vi "Experiment header-update fgv internal params.vi"(8 "error in (no error)":errorcluster, 10 "All header parameters in":T1={"LOGIN"={"User"="Olympus  20X", "Profile"="", "Software Version"="", "Experiment Date Time"=timestamp(0 s since 1904-01-01)}, "GLOBAL PARAMETERS"={"MicroscopeID"="", "Microscope Type"="", "Objective"="", "Field of View (um)"=0.0, "Fill time (us)"=0.0, "Experiment Type"=enum."In vivo", "Stimuli Trigger"=FALSE, "Speed Logging"=FALSE}, "IMAGING MODES"={"Time Series"=FALSE, "Motor Zstack"=FALSE, "AOL Zstack"=FALSE, "Functional Imaging"=FALSE, "Volume Imaging"=FALSE}, "TIME SERIES"={"Basic Image meta data"={"Wavelength (nm)"=0.0, "# averaged frames"=0.0, "laser power (%)"=0.0, "Pockels"=0.0, "pixel dwell time (us)"=0.0, "pmt 1"=0.0, "pmt 2"=0.0, "back apperture"=0.0, "zoom"=0.0, "field of view"=0.0, "Frame Size"=0, "AOL x centre"=0.0, "AOL y centre"=0.0, "Stage x position"=0.0, "Stage y position"=0.0, "Stage z position"=0.0}, "AOL z"=0.0}, "MOTOR Z-STACK "={"Hdr Basic Image meta data"={"Wavelength (nm)"=0.0, "# averaged frames"=0.0, "laser power (%)"=0.0, "Pockels"=0.0, "pixel dwell time (us)"=0.0, "pmt 1"=0.0, "pmt 2"=0.0, "back apperture"=0.0, "zoom"=0.0, "field of view"=0.0, "Frame Size"=0, "AOL x centre"=0.0, "AOL y centre"=0.0, "Stage x position"=0.0, "Stage y position"=0.0, "Stage z position"=0.0}, "Z Start"=0.0, "Z Stop"=0.0, "No of Planes"=0}, "AOL Z-STACK"={"Hdr Basic Image meta data"={"Wavelength (nm)"=0.0, "# averaged frames"=0.0, "laser power (%)"=0.0, "Pockels"=0.0, "pixel dwell time (us)"=0.0, "pmt 1"=0.0, "pmt 2"=0.0, "back apperture"=0.0, "zoom"=0.0, "field of view"=0.0, "Frame Size"=0, "AOL x centre"=0.0, "AOL y centre"=0.0, "Stage x position"=0.0, "Stage y position"=0.0, "Stage z position"=0.0}, "Z Start"=0.0, "Z Stop"=0.0, "No of Planes"=0}, "FUNCTIONAL IMAGING"={"Functional Mode"=enum."Point", "Pockels Modulation"=FALSE, "Number of pois"=0.0, "Number of miniscans"=0.0, "Number of cycles"=0.0, "Number of trials"=0.0, "Miniscan dwell time per pixel (us)"=0.0, "Number of pixels in miniscan"=0.0, "poi dwell time"=0.0, "Rectangle ROI length"=0.0, "Rectangle ROI height"=0.0, "AOL Mode"=enum."Raster", "Plane Mode"=0, "video length (sec)"=0.0, "Frame rate (fps)"=0.0, "Stimuli Timing (usec)"=0.0, "Acquisition Length"=0.0, "Basic Image meta data"={"Wavelength (nm)"=0.0, "# averaged frames"=0.0, "laser power (%)"=0.0, "Pockels"=0.0, "pixel dwell time (us)"=0.0, "pmt 1"=0.0, "pmt 2"=0.0, "back apperture"=0.0, "zoom"=0.0, "field of view"=0.0, "Frame Size"=0, "AOL x centre"=0.0, "AOL y centre"=0.0, "Stage x position"=0.0, "Stage y position"=0.0, "Stage z position"=0.0}, "Z Start (um)"=0.0, "Z Stop (um)"=0.0}, "VOLUME IMAGING"={"Functional Mode"=enum."Point", "Pockels Modulation"=FALSE, "Number of pois"=0.0, "Number of miniscans"=0.0, "Number of cycles"=0.0, "Number of trials"=0.0, "Miniscan dwell time per pixel (us)"=0.0, "Number of pixels in miniscan"=0.0, "poi dwell time"=0.0, "Rectangle ROI length"=0.0, "Rectangle ROI height"=0.0, "AOL Mode"=enum."Raster", "Plane Mode"=0, "video length (sec)"=0.0, "Frame rate (fps)"=0.0, "Stimuli Timing (usec)"=0.0, "Acquisition Length"=0.0, "Basic Image meta data"={"Wavelength (nm)"=0.0, "# averaged frames"=0.0, "laser power (%)"=0.0, "Pockels"=0.0, "pixel dwell time (us)"=0.0, "pmt 1"=0.0, "pmt 2"=0.0, "back apperture"=0.0, "zoom"=0.0, "field of view"=0.0, "Frame Size"=0, "AOL x centre"=0.0, "AOL y centre"=0.0, "Stage x position"=0.0, "Stage y position"=0.0, "Stage z position"=0.0}, "Z Start (um)"=0.0, "Z Stop (um)"=0.0}, "MOVEMENT CORRECTION"={"Movement Correction"=FALSE, "Axial Reference"=FALSE, "Reference X Pixels"=0.0, "Reference Y Pixels"=0.0, "Reference Source"=enum."Green channel", "Reference dwell time (us)"=0.0, "Number of Z lines"=0.0, "Size of Z pixels"=0.0, "Axial Pixels"=0.0, "Reference Zoom"=0.0, "Reference Average"=0.0, "Proportional Scale"=0.0, "Integral Scale"=0.0, "Proportional Scale Z"=0.0, "Integral Scale Z"=0.0, "Scan Interval"=0.0, "Ref Plot Refresh Rate"=0.0}, "CALIBRATION"={"Pockels Calibration File"=path "", "Calibration_ini file"=path "", "Setup_ini file"=path ""}, "STATISTICS"={"Z-stack duration (sec)"=0.0, "Number of acquired data-points"=0.0, "Acquisition time (ms)"=0.0, "Number of acquired frames"=0.0}, "BIOLOGY INFORMATION"={"Animal Code or Name"="", "Animal DoB"="", "Animal Age"="", "Animal Sex"="", "Animal Weight"="", "Date of Injection"="", "Date of Implant"="", "Site of Injection"="", "Animal Ear Notch"="", "AAV constructs"="", "Genetic background"="", "Optical reporter"="", "Region of brain imaged"="", "Other \ncomments"=""}} {"VOLUME IMAGING"."Plane Mode" items=["XY Plane", "XZ Plane", "YZ Plane", "arbitraryplane"]; "VOLUME IMAGING"."Basic Image meta data"."Frame Size" items=["100X100"=100, "128X128"=128, "200X200"=200, "256X256"=256, "512X512"=512, "1024x1024"=1024, "2048x2048"=2048]; "AOL Z-STACK"."Hdr Basic Image meta data"."Frame Size" items=["100X100"=100, "128X128"=128, "200X200"=200, "256X256"=256, "512X512"=512, "1024x1024"=1024, "2048x2048"=2048]; "MOTOR Z-STACK"."Hdr Basic Image meta data"."Frame Size" items=["100X100"=100, "128X128"=128, "200X200"=200, "256X256"=256, "512X512"=512, "1024x1024"=1024, "2048x2048"=2048]; "FUNCTIONAL IMAGING"."Plane Mode" items=["XY Plane", "XZ Plane", "YZ Plane", "arbitraryplane"]; "FUNCTIONAL IMAGING"."Basic Image meta data"."Frame Size" items=["100X100"=100, "128X128"=128, "200X200"=200, "256X256"=256, "512X512"=512, "1024x1024"=1024, "2048x2048"=2048]; "TIME SERIES"."Basic Image meta data"."Frame Size" items=["100X100"=100, "128X128"=128, "200X200"=200, "256X256"=256, "512X512"=512, "1024x1024"=1024, "2048x2048"=2048]}, 11 "All header parameters / Header module interface cluster":refnum<vi>) -> (0 "error out":errorcluster, 3 "All header parameters OUT":refnum<vi>)   [LabVIEW 2017]
uses:
  Typedefs/Header parameters cluster-ALL.ctl
  Typedefs/Header subclusters/Header params -Login.ctl
  Typedefs/Header subclusters/Header params-Global Parameters.ctl
  Misc/Experiment Type.ctl
  Typedefs/Header subclusters/Header params-Imaging Modes.ctl
  Typedefs/Header subclusters/Header params-Time Series.ctl
  Typedefs/Header subclusters/Header params-Basic image meta data.ctl
  Typedefs/Frame Size.ctl
  Typedefs/Header subclusters/Header params-Motor Z-stack.ctl
  Typedefs/Header subclusters/Header params-AOL Z-stack.ctl
  Typedefs/Header subclusters/Header params-Functional Imaging.ctl
  Typedefs/Functional Mode.ctl
  Typedefs/AOL modes.ctl
  Typedefs/Plane Mode.ctl
  Typedefs/Header subclusters/Header params-Movement correction.ctl
  Typedefs/Reference source.ctl
  Typedefs/Header subclusters/Header params-Calibration Setup.ctl
  Typedefs/Header subclusters/Header params-statistics.ctl
  Misc/Biology Information.ctl
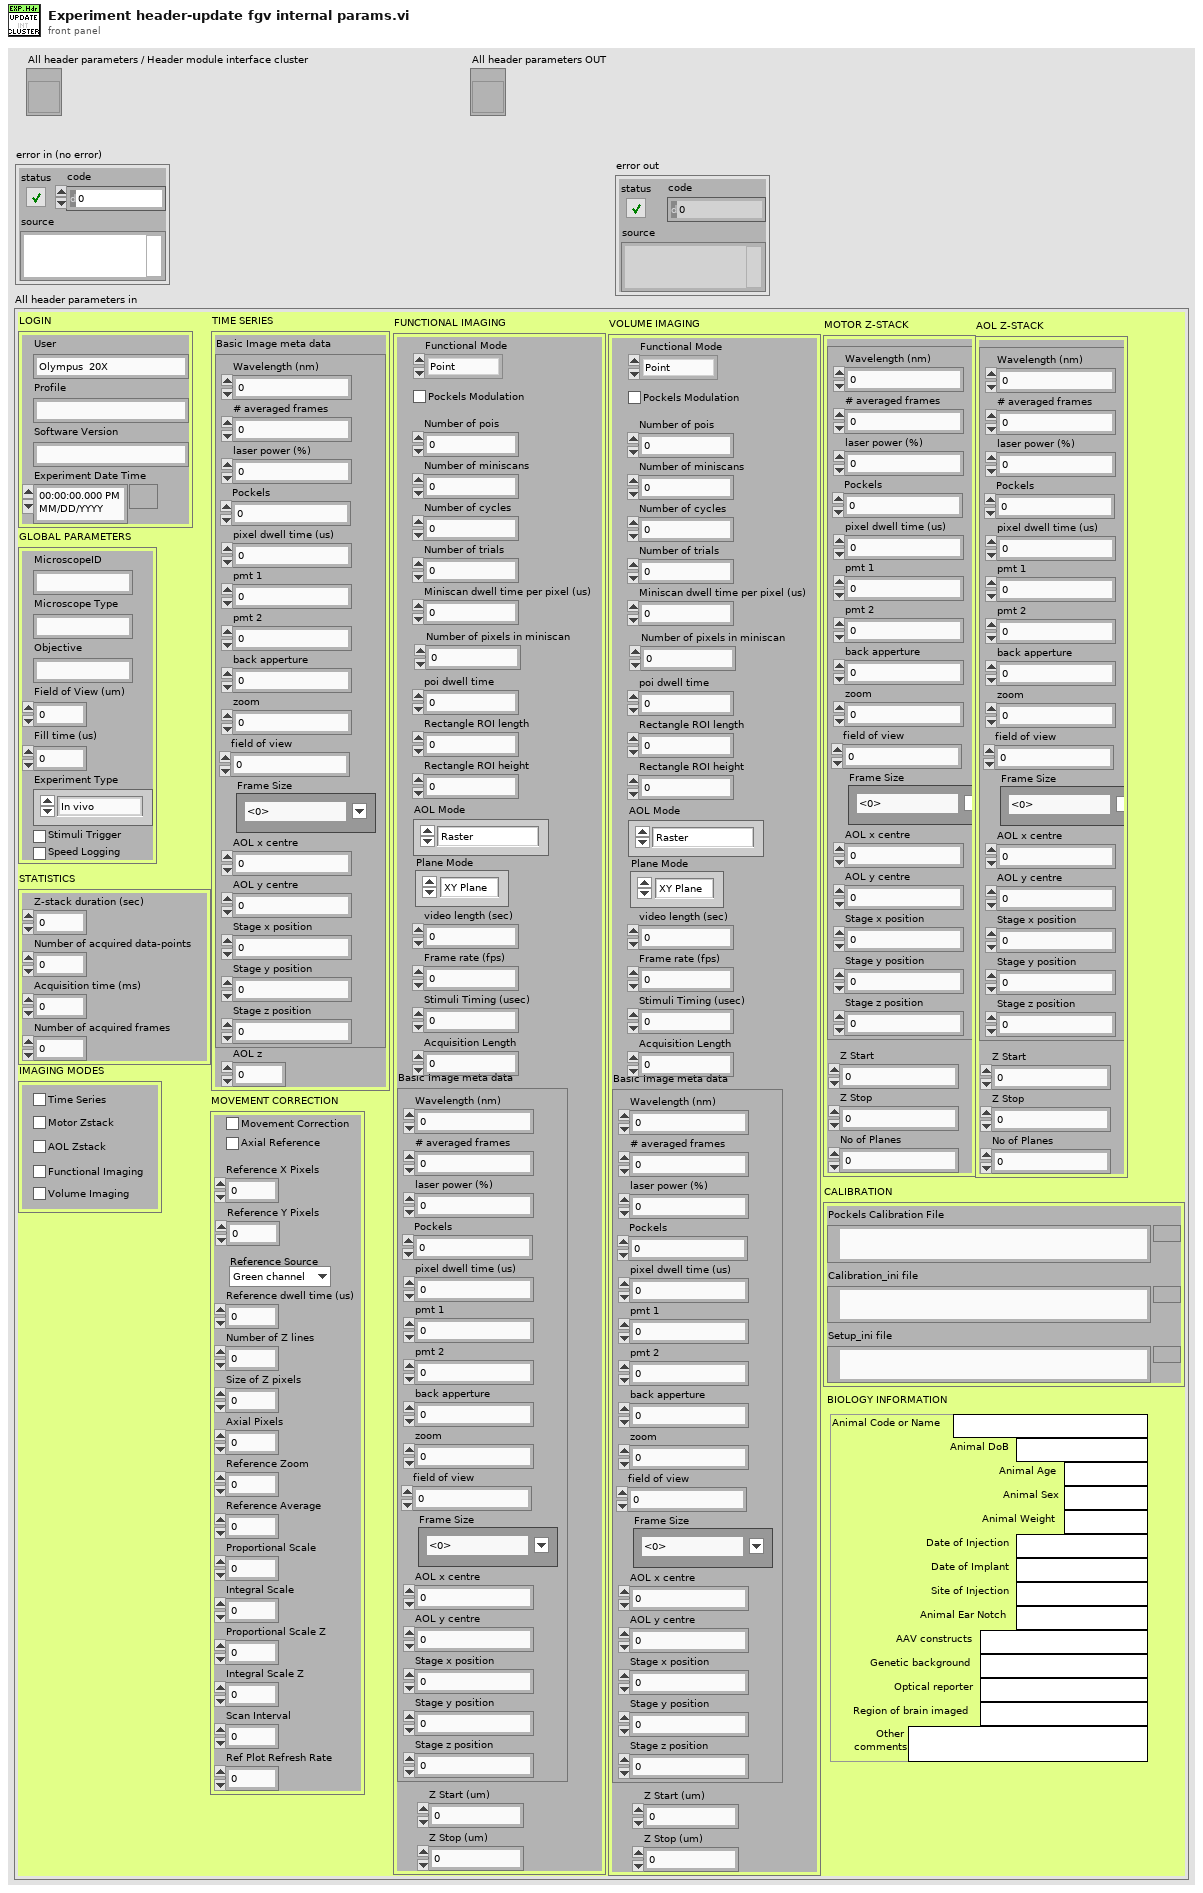
[diagram p1: front panel]
types:
  T1 = typedef "Header parameters cluster-ALL.ctl" = cluster{"LOGIN":T2, "GLOBAL PARAMETERS":T3, "IMAGING MODES":T5, "TIME SERIES":T6, "MOTOR Z-STACK ":T9, "AOL Z-STACK":T10, "FUNCTIONAL IMAGING":T11, "VOLUME IMAGING":T11, "MOVEMENT CORRECTION":T15, "CALIBRATION":T17, "STATISTICS":T18, "BIOLOGY INFORMATION":T19}
  T2 = typedef "Header params -Login.ctl" = cluster{"User":string, "Profile":string, "Software Version":string, "Experiment Date Time":timestamp}
  T3 = typedef "Header params-Global Parameters.ctl" = cluster{"MicroscopeID":string, "Microscope Type":string, "Objective":string, "Field of View (um)":dbl, "Fill time (us)":dbl, "Experiment Type":T4, "Stimuli Trigger":bool, "Speed Logging":bool}
  T4 = typedef "Experiment Type.ctl" = enum16{"In vivo", "In vitro", "Testing", "Calibration", "Other"}
  T5 = typedef "Header params-Imaging Modes.ctl" = cluster{"Time Series":bool, "Motor Zstack":bool, "AOL Zstack":bool, "Functional Imaging":bool, "Volume Imaging":bool}
  T6 = typedef "Header params-Time Series.ctl" = cluster{"Basic Image meta data":T7, "AOL z":dbl}
  T7 = typedef "Header params-Basic image meta data.ctl" = cluster{"Wavelength (nm)":dbl, "# averaged frames":dbl, "laser power (%)":dbl, "Pockels":dbl, "pixel dwell time (us)":dbl, "pmt 1":dbl, "pmt 2":dbl, "back apperture":dbl, "zoom":dbl, "field of view":dbl, "Frame Size":T8, "AOL x centre":dbl, "AOL y centre":dbl, "Stage x position":dbl, "Stage y position":dbl, "Stage z position":dbl}
  T8 = typedef "Frame Size.ctl" = u16
  T9 = typedef "Header params-Motor Z-stack.ctl" = cluster{"Hdr Basic Image meta data":T7, "Z Start":dbl, "Z Stop":dbl, "No of Planes":i32}
  T10 = typedef "Header params-AOL Z-stack.ctl" = cluster{"Hdr Basic Image meta data":T7, "Z Start":dbl, "Z Stop":dbl, "No of Planes":i32}
  T11 = typedef "Header params-Functional Imaging.ctl" = cluster{"Functional Mode":T12, "Pockels Modulation":bool, "Number of pois":dbl, "Number of miniscans":dbl, "Number of cycles":dbl, "Number of trials":dbl, "Miniscan dwell time per pixel (us)":dbl, "Number of pixels in miniscan":dbl, "poi dwell time":dbl, "Rectangle ROI length":dbl, "Rectangle ROI height":dbl, "AOL Mode":T13, "Plane Mode":T14, "video length (sec)":dbl, "Frame rate (fps)":dbl, "Stimuli Timing (usec)":dbl, "Acquisition Length":dbl, "Basic Image meta data":T7, "Z Start (um)":dbl, "Z Stop (um)":dbl}
  T12 = typedef "Functional Mode.ctl" = enum16{"Point", "Line", "Patch", "Plane", "Volume"}
  T13 = typedef "AOL modes.ctl" = enum16{"Raster", "Structural", "Pointing", "Mini Scan", "Alignment"}
  T14 = typedef "Plane Mode.ctl" = u16
  T15 = typedef "Header params-Movement correction.ctl" = cluster{"Movement Correction":bool, "Axial Reference":bool, "Reference X Pixels":dbl, "Reference Y Pixels":dbl, "Reference Source":T16, "Reference dwell time (us)":dbl, "Number of Z lines":dbl, "Size of Z pixels":dbl, "Axial Pixels":dbl, "Reference Zoom":dbl, "Reference Average":dbl, "Proportional Scale":dbl, "Integral Scale":dbl, "Proportional Scale Z":dbl, "Integral Scale Z":dbl, "Scan Interval":dbl, "Ref Plot Refresh Rate":dbl}
  T16 = typedef "Reference source.ctl" = enum16{"Green channel", "Red channel"}
  T17 = typedef "Header params-Calibration Setup.ctl" = cluster{"Pockels Calibration File":path, "Calibration_ini file":path, "Setup_ini file":path}
  T18 = typedef "Header params-statistics.ctl" = cluster{"Z-stack duration (sec)":dbl, "Number of acquired data-points":dbl, "Acquisition time (ms)":dbl, "Number of acquired frames":dbl}
  T19 = typedef "Biology Information.ctl" = cluster{"Animal Code or Name":string, "Animal DoB":string, "Animal Age":string, "Animal Sex":string, "Animal Weight":string, "Date of Injection":string, "Date of Implant":string, "Site of Injection":string, "Animal Ear Notch":string, "AAV constructs":string, "Genetic background":string, "Optical reporter":string, "Region of brain imaged":string, "Other \ncomments":string}
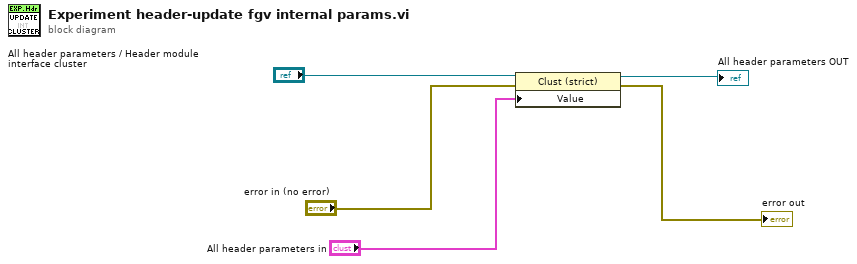
[diagram p0: block diagram]
diagram:
  n1 = property class="Clust (strict)"(reference="All header parameters / Header module interface cluster", error in="error in (no error)", "Value"="All header parameters in") -> (reference out=→"All header parameters OUT":refnum<vi>, error out=→"error out":errorcluster)
